vi "CalculateBounds.vi"(8 "error in (no error)":errorcluster, 11 "menu in":refnum<class "menu.lvclass">) -> (0 "error out":errorcluster, 2 "bounds":cluster{"width":u32, "height":u32}, 3 "menu out":refnum<class "menu.lvclass">)   [LabVIEW 2009, in "menu.lvclass"]
uses:
  menu.lvclass
  menu.lvclass/menu.ctl
  Menu Item/menu item.lvclass
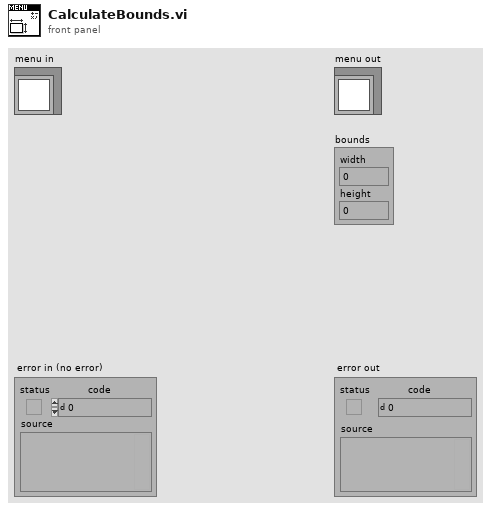
[diagram p1: front panel]
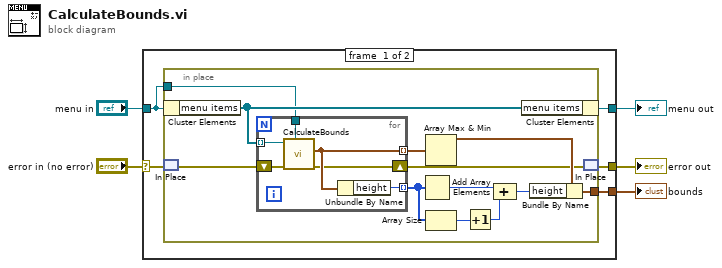
[diagram p0: block diagram]
diagram:
  n1 = case shown="No Error" "error in (no error)" {
    selector: "error in (no error)" -> [w8 w30]
    tunnel: [w7 w30] -> w3
    tunnel: [w10 w29] -> w5
    tunnel: "menu in" -> [w9 w29]
    tunnel: [w6 _] -> w1
    frame #0 {
      n2 = in-place {
        in-place-border: w9 -> [w14]
        in-place-border: [w11] -> w6
        n3 = in-place-cluster #1(w9) -> ("menu items"=w15:refnum<class "menu item.lvclass">[])
        n4 = in-place-match #2(w8) -> (w13:errorcluster)
        n5 = for {
          tunnel: w15 -> [w28] mode=indexing
          tunnel: [w27] -> w22 mode=indexing
          tunnel: [w26] -> w20 mode=indexing
          shift-right: [w24] -> w12
          shift-left: w13 -> [w25]
          tunnel: w14 -> [w23]
          n6 = call-dynamic "CalculateBounds.vi"("menu in"=w23, "error in (no error)"=w25, "menu item in"=w28) -> ("error out"=w24:errorcluster, "bounds"=w27:cluster{"width":u32, "height":u32})  [unwired: 6 in, 1 out]
          n7 = Unbundle By Name(w27) -> ("height"=w26:u32)
        }
        n8 = Add Array Elements(numeric array=w20) -> (sum=w18:u32)
        n9 = Array Max & Min(array=w22) -> (max value=w21:cluster{"width":u32, "height":u32})  [unwired: 3 out]
        n10 = Array Size(array=w20) -> (size(s)=w19:i32)
        n11 = Increment(x=w19) -> (x+1=w17:i32)
        n12 = Compound Arithmetic op=ADD(w18, w17) -> (w16:u32)
        n13 = in-place-cluster #1("menu items"=w15) -> (w10:refnum<class "menu.lvclass">)
        n14 = Bundle By Name(cluster=w21, "height"=w16) -> (w11:cluster{"width":u32, "height":u32})
        n15 = in-place-match #2(w12) -> (w7:errorcluster)
      }
    }
    frame #1 {
    }
  }
  "menu out" <- w5
  "error out" <- w3
  "bounds" <- w1
